vi "3D Axis Rendering.vi"(11 "rotation matrix":T29=[[1.0, 0.0, 0.0, 1.0], [0.0, 1.0, 0.0, 0.0], [0.0, 0.0, 1.0, 0.0], [0.0, 0.0, 0.0, 1.0]]) -> (3 "SceneNode out":refnum<vi>(3d-picture))   [LabVIEW 2017]
uses:
  <vilib>/Analysis/Matrix/Datatypes/RealMatrix.ctl
  <vilib>/Math Plots/3D Math Plots/3D Plot/3D Plot/Typedef/Property Cluster.ctl
  <vilib>/Math Plots/3D Math Plots/3D Plot/3D Plot/Typedef/Graph Property.ctl
  <vilib>/Math Plots/3D Math Plots/3D Plot/3D Plot/Typedef/General Property.ctl
  <vilib>/Math Plots/3D Math Plots/3D Plot/3D Plot/Typedef/View Property.ctl
  <vilib>/Math Plots/3D Math Plots/3D Plot/3D Plot/Typedef/Grid Plane.ctl
  <vilib>/Math Plots/3D Math Plots/3D Plot/3D Plot/Typedef/Light Property.ctl
  <vilib>/Math Plots/3D Math Plots/3D Plot/3D Plot/Typedef/Light Specific.ctl
  <vilib>/Math Plots/3D Math Plots/3D Plot/3D Plot/Typedef/Axis Property.ctl
  <vilib>/Math Plots/3D Math Plots/3D Plot/3D Plot/Typedef/Caption Property.ctl
  <vilib>/Math Plots/3D Math Plots/3D Plot/3D Plot/Typedef/Label Property.ctl
  <vilib>/Math Plots/3D Math Plots/3D Plot/3D Plot/Typedef/Range Property.ctl
  <vilib>/Math Plots/3D Math Plots/3D Plot/3D Plot/Typedef/Range Clusters.ctl
  <vilib>/Math Plots/3D Math Plots/3D Plot/3D Plot/Typedef/Grid Property.ctl
  <vilib>/Math Plots/3D Math Plots/3D Plot/3D Plot/Typedef/Tick Property.ctl
  <vilib>/Math Plots/3D Math Plots/3D Plot/3D Plot/Typedef/Value Pair Property.ctl
  <vilib>/Math Plots/3D Math Plots/3D Plot/3D Plot/Typedef/Value Pair Cluster.ctl
  <vilib>/Math Plots/3D Math Plots/3D Plot/3D Plot/Typedef/Format Property.ctl
  <vilib>/Math Plots/3D Math Plots/3D Plot/3D Plot/Typedef/Cursor Property Array.ctl
  <vilib>/Math Plots/3D Math Plots/3D Plot/3D Plot/Typedef/Cursor Property.ctl
  <vilib>/Math Plots/3D Math Plots/3D Plot/3D Plot/Typedef/Cursor Position.ctl
  <vilib>/Math Plots/3D Math Plots/3D Plot/3D Plot/Typedef/Cursor Point.ctl
  <vilib>/Math Plots/3D Math Plots/3D Plot/3D Plot/Typedef/Sprite Type.ctl
  <vilib>/Math Plots/3D Math Plots/3D Plot/3D Plot/Typedef/Cursor Line.ctl
  <vilib>/Math Plots/3D Math Plots/3D Plot/3D Plot/Typedef/Line Type.ctl
  <vilib>/Math Plots/3D Math Plots/3D Plot/3D Plot/Typedef/Cursor Plane.ctl
  <vilib>/Math Plots/3D Math Plots/3D Plot/3D Plot/Typedef/Cursor Text.ctl
  <vilib>/Math Plots/3D Math Plots/3D Plot/3D Plot/Typedef/Apearance Property.ctl
  <vilib>/Math Plots/3D Math Plots/3D Plot/3D Plot/Typedef/Item Visibility.ctl
  <vilib>/Math Plots/3D Math Plots/3D Plot/3D Plot/Typedef/Actual Transform.ctl
  <vilib>/picture/3D Picture Control/Object/Add Object (reference).vi
  <vilib>/picture/3D Picture Control/Object/Add Object (no reference).vi
  <vilib>/picture/3D Picture Control/Object/Create Object (name).vi
  <vilib>/picture/3D Picture Control/NI_3D Picture Control.lvlib
  <vilib>/Math Plots/3D Math Plots/3D Plot/3D Plot/3D Plot.lvclass
  <vilib>/robotics/Kinematics/NI_Kinematics.lvlib
  <vilib>/Analysis/Matrix/NI_Matrix.lvlib
panel:
  in  "Property Cluster":T1={"Graph Property"={"General Property"={"Plot Area Color"=16448250, "Fast Draw?"=TRUE, "Clip Data?"=FALSE}, "View Property"={"Projection Mode"=enum."Orthographic", "View Direction"=enum."User Defined", "User Defined View Direction"={"View Latitude"=1.0472, "View Longitude"=0.7853981, "View Distance"=2.0}}, "Grid Plane"={"Grid Plane Visible"={"Draw Grid Plane X-Y"=TRUE, "Draw Grid Plane Y-Z"=TRUE, "Draw Grid Plane X-Z"=TRUE}, "Grid Antialiasing"=TRUE, "Grid Frame Color"=0}}, "Light Property"={"Enable Lighting?"=TRUE, "Ambient Color"=16448250, "Light Array"=[{"Enable Light?"=TRUE, "Light Color"=16448250, "Light Latitude"=0.7853981, "Light Longitude"=0.7853981, "Light Distance"=10.0, "Attenuation"=enum."None"}, {"Enable Light?"=FALSE, "Light Color"=16448250, "Light Latitude"=0.785398, "Light Longitude"=0.785398, "Light Distance"=10.0, "Attenuation"=enum."None"}, {"Enable Light?"=FALSE, "Light Color"=16448250, "Light Latitude"=0.785398, "Light Longitude"=0.785398, "Light Distance"=10.0, "Attenuation"=enum."None"}, {"Enable Light?"=FALSE, "Light Color"=16448250, "Light Latitude"=0.785398, "Light Longitude"=0.785398, "Light Distance"=10.0, "Attenuation"=enum."None"}]}, "Axis Property"={"Caption Property"={"Show Caption"={"Show Normal X Caption"=TRUE, "Show Normal Y Caption"=TRUE, "Show Normal Z Caption"=TRUE, "Show Opposite X Caption"=TRUE, "Show Opposite Y Caption"=TRUE, "Show Opposite Z Caption"=TRUE}, "Caption Color"={"Caption Color X"=0, "Caption Color Y"=0, "Caption Color Z"=0}, "Caption Size"={"Caption Size X"=12, "Caption Size Y"=12, "Caption Size Z"=12}, "Caption String"={"Caption X"="X Axis", "Caption Y"="Y Axis", "Caption Z "="Z Axis"}}, "Label Property"={"Show Label"={"Show Normal X Label"=TRUE, "Show Normal Y Label"=TRUE, "Show Normal Z Label"=TRUE, "Show Opposite X Label"=TRUE, "Show Opposite Y Label"=TRUE, "Show Opposite Z Label"=TRUE}, "Label Color"={"Label Color X"=0, "Label Color Y"=0, "Label Color Z"=0}, "Label Size"={"Label Size X"=8, "Label Size Y"=8, "Labe Size Z"=8}}, "Range Property"={"Range Cluster"={"X Range"={"Max X"=10.0, "Min X"=0.0}, "Y Range"={"Max Y"=10.0, "Min Y"=0.0}, "Z Range"={"Max Z"=10.0, "Min Z"=0.0}}, "Auto Range"={"Auto Range X"=TRUE, "Auto Range Y"=TRUE, "Auto Range Z"=TRUE}, "Inverted"={"Inverted X"=FALSE, "Inverted Y"=FALSE, "Inverted Z"=FALSE}, "Logarithm"={"Logarithm X"=FALSE, "Logarithm Y"=FALSE, "Logarithm Z"=FALSE}}, "Grid Property"={"Major Grid Visible"={"Draw Major Grid X"=TRUE, "Draw Major Grid Y"=TRUE, "Draw Major Grid Z"=TRUE}, "Major Grid Color"={"Major Grid Color X"=0, "Major Grid Color Y"=0, "Major Grid Color Z"=0}, "Minor Grid Visible"={"Draw Minor Grid X"=FALSE, "Draw Minor Grid Y"=FALSE, "Draw Minor Grid Z"=FALSE}, "Minor Grid Color"={"Minor Grid Color X"=9868950, "Minor Grid Color Y"=9868950, "Minor Grid Color Z"=9868950}}, "Ticks Property"={"Major Tick Visible"={"Draw Major Tick X"=TRUE, "Draw Major Tick Y"=TRUE, "Draw Major Tick Z"=TRUE}, "Major Tick Color"={"Major Tick Color X"=0, "Major Tick Color Y"=0, "Major Tick Color Z"=0}, "Major Count"={"Major Count X"=5, "Major Count Y"=5, "Major Count Z"=5}, "Minor Tick Visible"={"Draw Minor Tick X"=TRUE, "Draw Minor Tick Y"=TRUE, "Draw Minor Tick Z"=TRUE}, "Minor Tick Color"={"Minor Tick Color X"=0, "Minor Tick Color Y"=0, "Minor Tick Color Z"=0}, "Minor Count"={"Minor Count X"=3, "Minor Count Y"=3, "Minor Count Z"=3}}}, "Value Pair Property"=[{"Value Pair Array"=[], "Show Tick"=FALSE, "Show Grid"=FALSE, " Label Mode"=enum."Name"}, {"Value Pair Array"=[], "Show Tick"=FALSE, "Show Grid"=FALSE, " Label Mode"=enum."Name"}, {"Value Pair Array"=[], "Show Tick"=FALSE, "Show Grid"=FALSE, " Label Mode"=enum."Name"}], "Format Property"=["%#.2g", "%#.2g", "%#.2g"], "Cursor Property Array"=[], "Appearance Property"={"Visibility"={"Projection Palette"=TRUE, "Color Ramp Palette"=TRUE}, "Active Index"={"Active Plot"=0, "Active Cursor"=0, "Active Axis"=enum."X-axis", "Active Value Pair"=enum."X-axis", "Active Light"=enum."Light 0"}, "Backup Data"={"Plot Name"=[]}}}
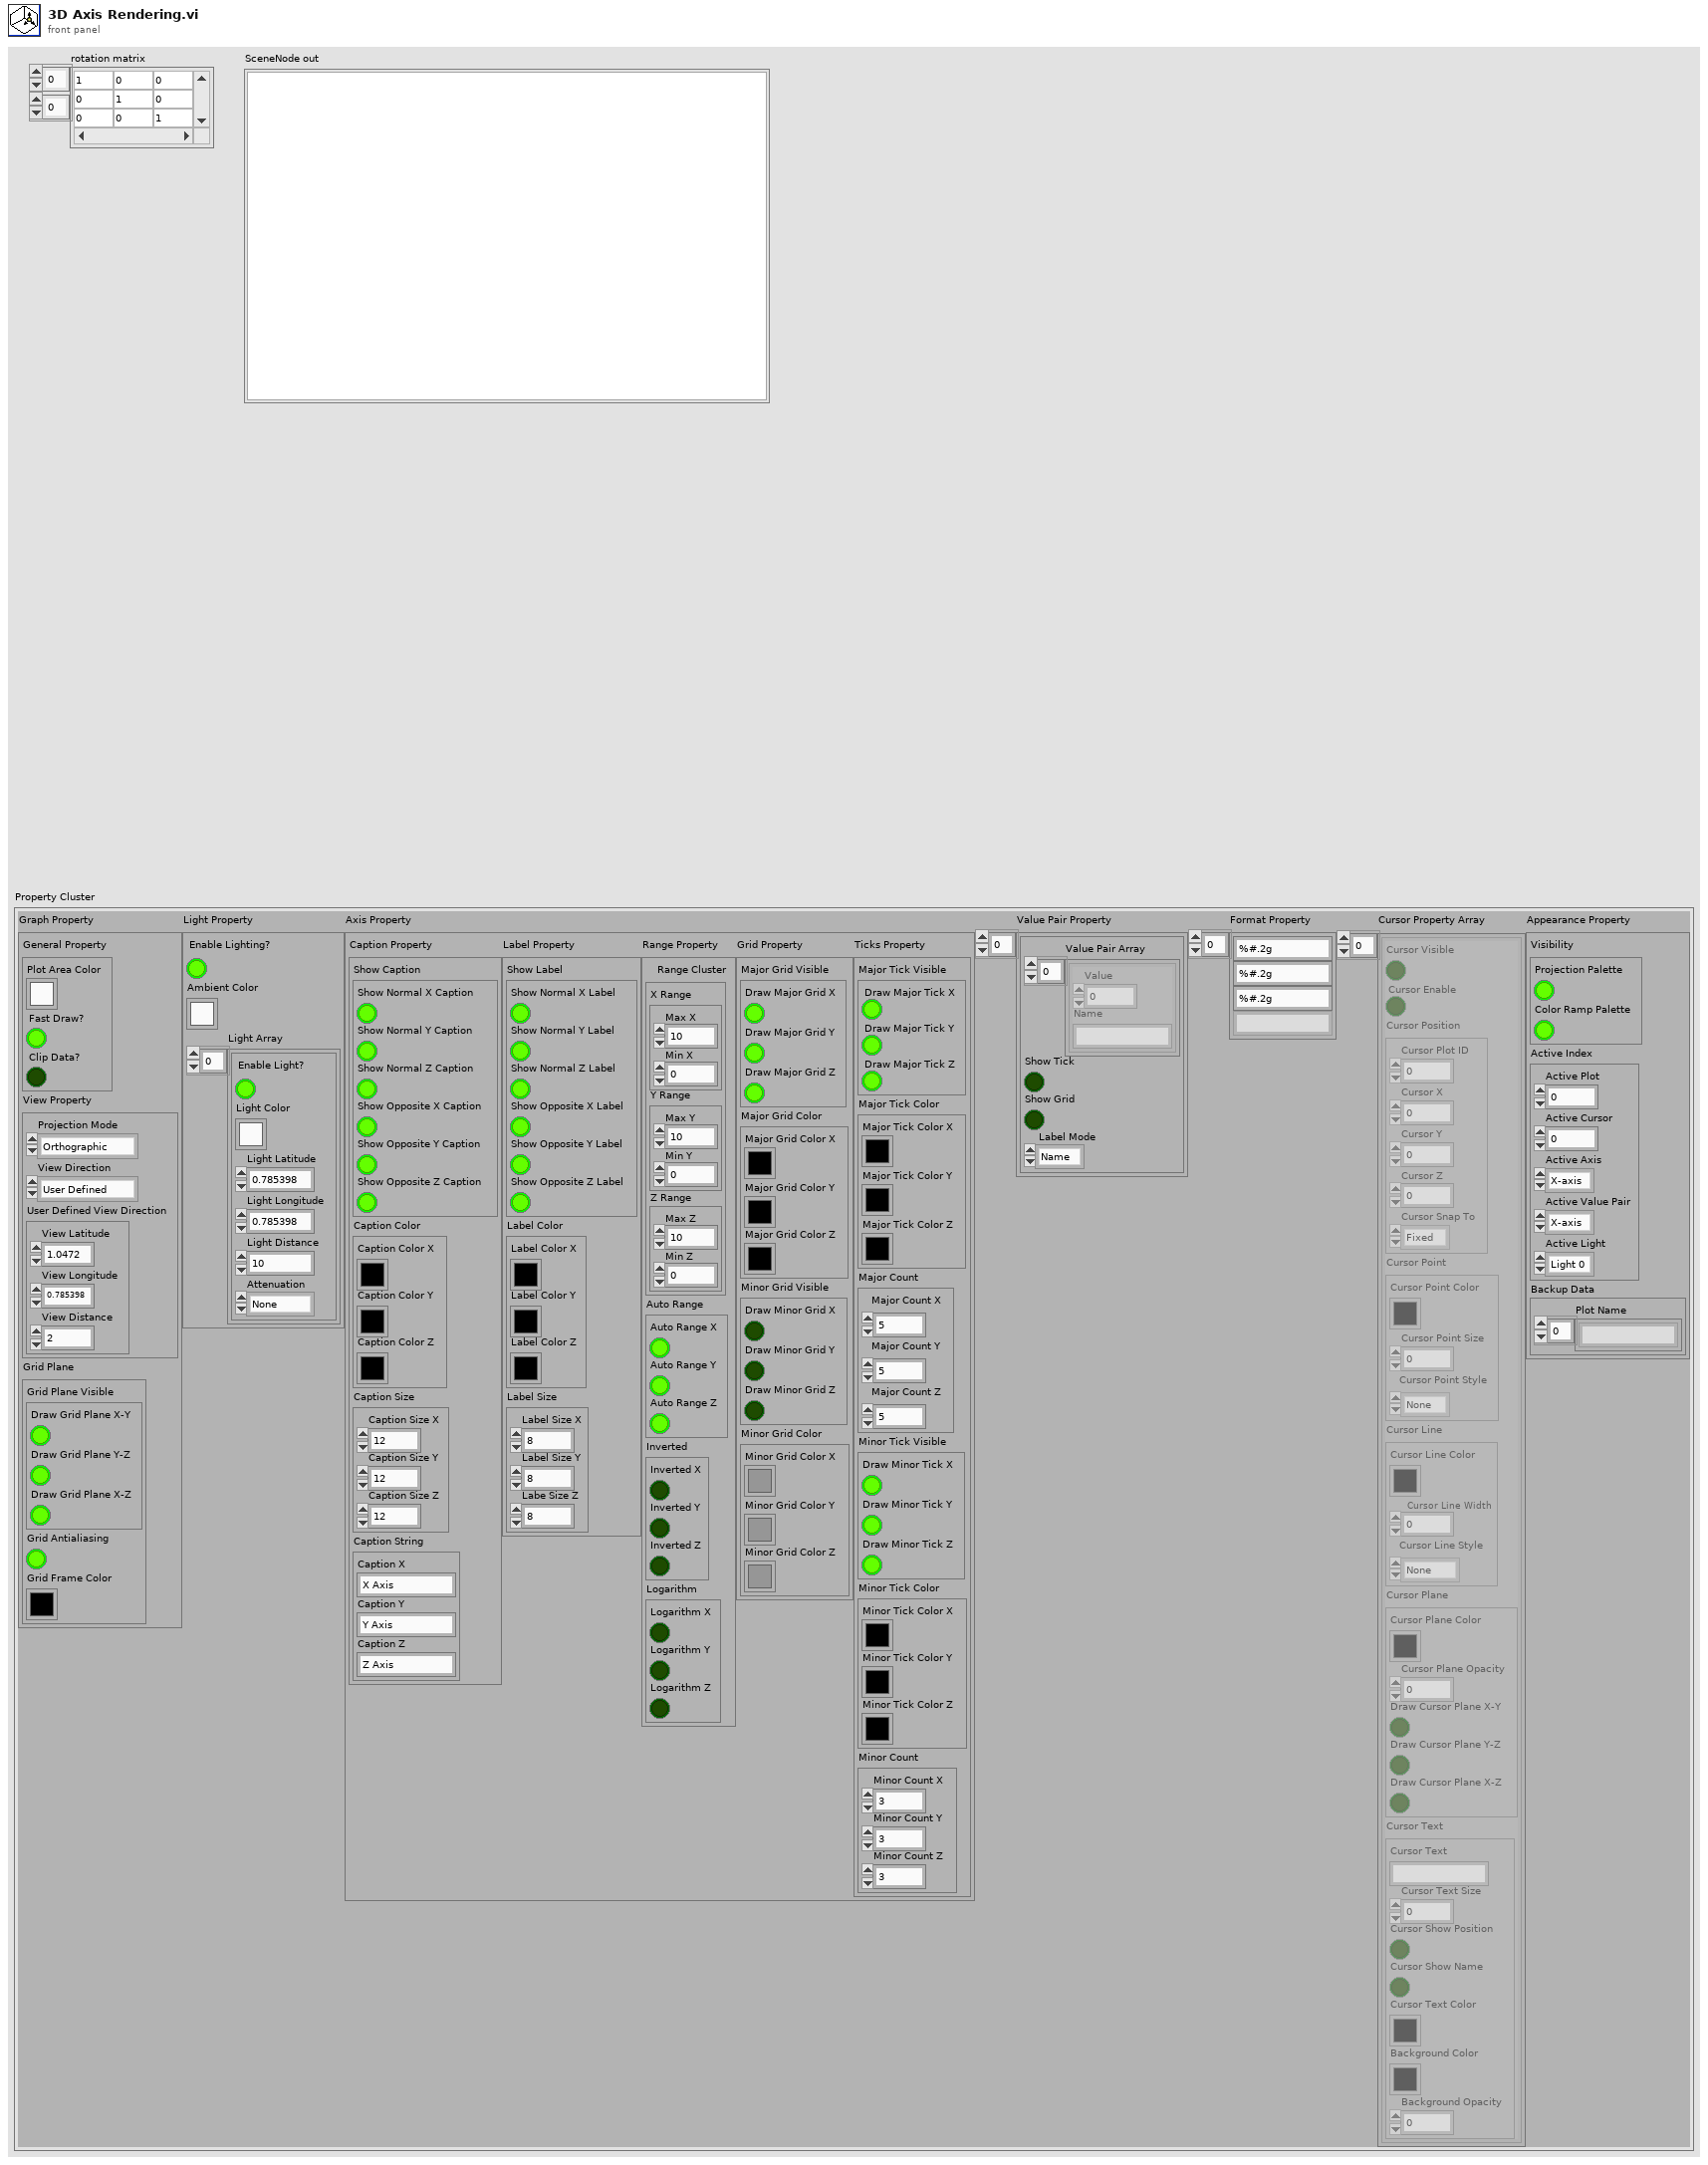
[diagram p1: front panel]
types:
  T1 = typedef "3D Plot.lvclass/Property Cluster.ctl" = cluster{"Graph Property":T2, "Light Property":T6, "Axis Property":T8, "Value Pair Property":T15, "Format Property":T17, "Cursor Property Array":T18, "Appearance Property":T27}
  T2 = typedef "3D Plot.lvclass/Graph Property.ctl" = cluster{"General Property":T3, "View Property":T4, "Grid Plane":T5}
  T3 = typedef "3D Plot.lvclass/General Property.ctl" = cluster{"Plot Area Color":u32, "Fast Draw?":bool, "Clip Data?":bool}
  T4 = typedef "3D Plot.lvclass/View Property.ctl" = cluster{"Projection Mode":enum16{"Orthographic", "Perspective"}, "View Direction":enum32{"Towards X-Y Plane", "Towards X-Z Plane", "Towards Y-Z Plane", "User Defined"}, "User Defined View Direction":cluster{"View Latitude":sgl, "View Longitude":sgl, "View Distance":sgl}}
  T5 = typedef "3D Plot.lvclass/Grid Plane.ctl" = cluster{"Grid Plane Visible":cluster{"Draw Grid Plane X-Y":bool, "Draw Grid Plane Y-Z":bool, "Draw Grid Plane X-Z":bool}, "Grid Antialiasing":bool, "Grid Frame Color":u32}
  T6 = typedef "3D Plot.lvclass/Light Property.ctl" = cluster{"Enable Lighting?":bool, "Ambient Color":u32, "Light Array":T7[]}
  T7 = typedef "3D Plot.lvclass/Light Specific.ctl" = cluster{"Enable Light?":bool, "Light Color":u32, "Light Latitude":sgl, "Light Longitude":sgl, "Light Distance":sgl, "Attenuation":enum16{"None", "Linear", "Quadratic"}}
  T8 = typedef "3D Plot.lvclass/Axis Property.ctl" = cluster{"Caption Property":T9, "Label Property":T10, "Range Property":T11, "Grid Property":T13, "Ticks Property":T14}
  T9 = typedef "3D Plot.lvclass/Caption Property.ctl" = cluster{"Show Caption":cluster{"Show Normal X Caption":bool, "Show Normal Y Caption":bool, "Show Normal Z Caption":bool, "Show Opposite X Caption":bool, "Show Opposite Y Caption":bool, "Show Opposite Z Caption":bool}, "Caption Color":cluster{"Caption Color X":u32, "Caption Color Y":u32, "Caption Color Z":u32}, "Caption Size":cluster{"Caption Size X":u16, "Caption Size Y":u16, "Caption Size Z":u16}, "Caption String":cluster{"Caption X":string, "Caption Y":string, "Caption Z ":string}}
  T10 = typedef "3D Plot.lvclass/Label Property.ctl" = cluster{"Show Label":cluster{"Show Normal X Label":bool, "Show Normal Y Label":bool, "Show Normal Z Label":bool, "Show Opposite X Label":bool, "Show Opposite Y Label":bool, "Show Opposite Z Label":bool}, "Label Color":cluster{"Label Color X":u32, "Label Color Y":u32, "Label Color Z":u32}, "Label Size":cluster{"Label Size X":u16, "Label Size Y":u16, "Labe Size Z":u16}}
  T11 = typedef "3D Plot.lvclass/Range Property.ctl" = cluster{"Range Cluster":T12, "Auto Range":cluster{"Auto Range X":bool, "Auto Range Y":bool, "Auto Range Z":bool}, "Inverted":cluster{"Inverted X":bool, "Inverted Y":bool, "Inverted Z":bool}, "Logarithm":cluster{"Logarithm X":bool, "Logarithm Y":bool, "Logarithm Z":bool}}
  T12 = typedef "3D Plot.lvclass/Range Clusters.ctl" = cluster{"X Range":cluster{"Max X":sgl, "Min X":sgl}, "Y Range":cluster{"Max Y":sgl, "Min Y":sgl}, "Z Range":cluster{"Max Z":sgl, "Min Z":sgl}}
  T13 = typedef "3D Plot.lvclass/Grid Property.ctl" = cluster{"Major Grid Visible":cluster{"Draw Major Grid X":bool, "Draw Major Grid Y":bool, "Draw Major Grid Z":bool}, "Major Grid Color":cluster{"Major Grid Color X":u32, "Major Grid Color Y":u32, "Major Grid Color Z":u32}, "Minor Grid Visible":cluster{"Draw Minor Grid X":bool, "Draw Minor Grid Y":bool, "Draw Minor Grid Z":bool}, "Minor Grid Color":cluster{"Minor Grid Color X":u32, "Minor Grid Color Y":u32, "Minor Grid Color Z":u32}}
  T14 = typedef "3D Plot.lvclass/Tick Property.ctl" = cluster{"Major Tick Visible":cluster{"Draw Major Tick X":bool, "Draw Major Tick Y":bool, "Draw Major Tick Z":bool}, "Major Tick Color":cluster{"Major Tick Color X":u32, "Major Tick Color Y":u32, "Major Tick Color Z":u32}, "Major Count":cluster{"Major Count X":u16, "Major Count Y":u16, "Major Count Z":u16}, "Minor Tick Visible":cluster{"Draw Minor Tick X":bool, "Draw Minor Tick Y":bool, "Draw Minor Tick Z":bool}, "Minor Tick Color":cluster{"Minor Tick Color X":u32, "Minor Tick Color Y":u32, "Minor Tick Color Z":u32}, "Minor Count":cluster{"Minor Count X":u16, "Minor Count Y":u16, "Minor Count Z":u16}}
  T15 = typedef "3D Plot.lvclass/Value Pair Property.ctl" = T16[]
  T16 = typedef "3D Plot.lvclass/Value Pair Cluster.ctl" = cluster{"Value Pair Array":cluster{"Value":sgl, "Name":string}[], "Show Tick":bool, "Show Grid":bool, " Label Mode":enum16{"Name", "Value", "None"}}
  T17 = typedef "3D Plot.lvclass/Format Property.ctl" = string[]
  T18 = typedef "3D Plot.lvclass/Cursor Property Array.ctl" = T19[]
  T19 = typedef "3D Plot.lvclass/Cursor Property.ctl" = cluster{"Cursor Visible":bool, "Cursor Enable":bool, "Cursor Position":T20, "Cursor Point":T21, "Cursor Line":T23, "Cursor Plane":T25, "Cursor Text":T26}
  T20 = typedef "3D Plot.lvclass/Cursor Position.ctl" = cluster{"Cursor Plot ID":i32, "Cursor X":sgl, "Cursor Y":sgl, "Cursor Z":sgl, "Cursor Snap To":enum16{"Fixed", "Nearest Plot", "Snap to Plot"}}
  T21 = typedef "3D Plot.lvclass/Cursor Point.ctl" = cluster{"Cursor Point Color":u32, "Cursor Point Size":sgl, "Cursor Point Style":T22}
  T22 = typedef "3D Plot.lvclass/Sprite Type.ctl" = enum16{"None", "Empty Square", "Solid Square", "Empty Diamond", "Solid Diamond", "Empty Circle", "Solid Circle", "Asterisk", "Bold X", "Wireframe Sphere", "Solid Sphere", "Wireframe Cube", "Solid Cube"}
  T23 = typedef "3D Plot.lvclass/Cursor Line.ctl" = cluster{"Cursor Line Color":u32, "Cursor Line Width":sgl, "Cursor Line Style":T24}
  T24 = typedef "3D Plot.lvclass/Line Type.ctl" = enum16{"None", "Solid", "Dash", "Dot", "Dash Dot"}
  T25 = typedef "3D Plot.lvclass/Cursor Plane.ctl" = cluster{"Cursor Plane Color":u32, "Cursor Plane Opacity":sgl, "Draw Cursor Plane X-Z":bool, "Draw Cursor Plane Y-Z":bool, "Draw Cursor Plane X-Y":bool}
  T26 = typedef "3D Plot.lvclass/Cursor Text.ctl" = cluster{"Cursor Text":string, "Cursor Text Size":u16, "Cursor Show Position":bool, "Cursor Show Name":bool, "Cursor Text Color":u32, "Background Color":u32, "Background Opacity":sgl}
  T27 = typedef "3D Plot.lvclass/Apearance Property.ctl" = cluster{"Visibility":T28, "Active Index":cluster{"Active Plot":i32, "Active Cursor":i32, "Active Axis":enum16{"X-axis", "Y-axis", "Z-axis"}, "Active Value Pair":enum16{"X-axis", "Y-axis", "Z-axis"}, "Active Light":enum16{"Light 0", "Light 1", "Light 2", "Light 3"}}, "Backup Data":cluster{"Plot Name":string[]}}
  T28 = typedef "3D Plot.lvclass/Item Visibility.ctl" = cluster{"Projection Palette":bool, "Color Ramp Palette":bool}
  T29 = typedef "NI_Matrix.lvlib/RealMatrix.ctl" = dbl[][]
  T30 = typedef "3D Plot.lvclass/Actual Transform.ctl" = cluster{"Scale Cluster":cluster{"X Scale":sgl, "Y Scale":sgl, "Z Scale":sgl}, "Translate Cluster":cluster{"X Translate":sgl, "Y Translate":sgl, "Z Translate":sgl}, "Actual Range":T12}
  T31 = typedef "3D Plot.lvclass/Object Cluster.ctl" = cluster{"Root Scene Object":refnum<vi>, "Fast Root Scene Object":refnum<vi>}
  T32 = cluster{"Z Translate":sgl, "Z Translate":sgl, "Z Translate":sgl}
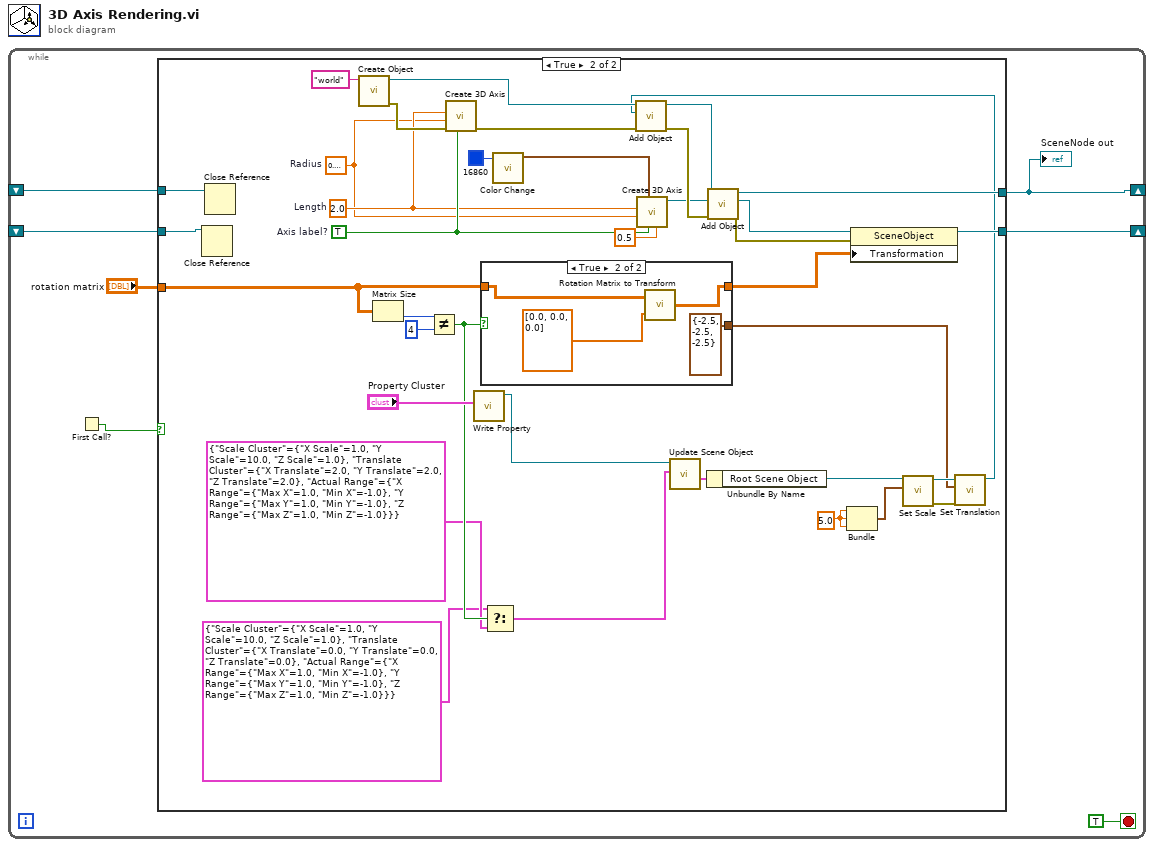
[diagram p0: block diagram]
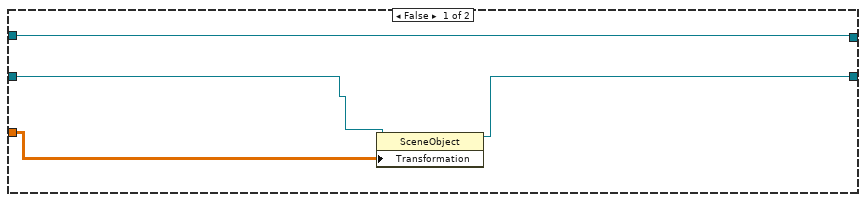
[diagram p2: hidden frame]
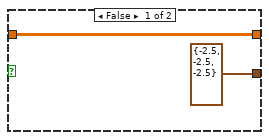
[diagram p3: hidden frame]
diagram:
  n1 = while {
    shift-right: [w5] -> _
    shift-left: _ -> [w2]
    shift-right: [w4] -> _
    shift-left: _ -> [w3]
    stop <- TRUE stop-if-true
    n2 = First Call?() -> (First Call?: T/F=w1:bool)
    n3 = case shown="True" w1 {
      tunnel: [w11 w40] -> w4
      tunnel: [w9 w27] -> w5
      tunnel: "rotation matrix" -> [w8 w23]
      tunnel: w3 -> [w11 w13]
      tunnel: w2 -> [w10 w12]
      frame False {
        n4 = property class="SceneObject"(reference=w10, "Transformation"=w8) -> (reference out=w9:refnum<vi>)  [unwired: 1 in, 1 out]
      }
      frame True {
        w33 = sgl 5.0 ("Z Translate")
        w42 = sgl 2.0  # Length
        w41 = sgl 0.1  # Radius
        w48 = TRUE  # Axis label?
        n5 = Close Reference(reference=w12) -> ()  [unwired: 1 in, 1 out]
        n6 = Close Reference(reference=w13) -> ()  [unwired: 1 in, 1 out]
        n7 = call-poly <vilib>:"Create Object.vi"("Name"="world") -> ("error out"=w44:errorcluster, "Scene:New Object"=w37:refnum<vi>)  [unwired: 9 in]
        n8 = Matrix Size(0:w23) -> (2:w25:i32)  [unwired: 1 out]
        n9 = Not Equal?(x=w25, y=4) -> (x != y?=w22:bool)
        n10 = call <vilib>:"Create 3D Axis.vi"("Axis label?"=w48, "error in (no error)"=w44, "Radius"=w41, "Length"=w42) -> ("error out"=w36:errorcluster)  [unwired: 6 in, 1 out]
        n11 = call <vilib>:"Write Property.vi"("Property Cluster"="Property Cluster") -> ("3D Plot.lvclass out"=w29:refnum<class "3D Plot.lvclass">)  [unwired: 9 in, 1 out]
        n12 = case shown="True" w22 {
          tunnel: w23 -> [w49 w54]
          tunnel: [w49 w53] -> w14
          tunnel: [cluster{"X":sgl, "Y":sgl, "Z":sgl} {"X"=-2.5, "Y"=-2.5, "Z"=-2.5} ("Translation") cluster{"X":sgl, "Y":sgl, "Z":sgl} {"X"=-2.5, "Y"=-2.5, "Z"=-2.5} ("Translation")] -> w15
          frame False {
          }
          frame True {
            n13 = call <vilib>:"Rotation Matrix to Transform.vi"("translation vector"=dbl[] [0.0, 0.0, 0.0], "rotation matrix"=w54) -> ("transform"=w53:T29)
          }
        }
        n14 = Select(t=T30 {"Scale Cluster"={"X Scale"=1.0, "Y Scale"=10.0, "Z Scale"=1.0}, "Translate Cluster"={"X Translate"=0.0, "Y Translate"=0.0, "Z Translate"=0.0}, "Actual Range"={"X Range"={"Max X"=1.0, "Min X"=-1.0}, "Y Range"={"Max Y"=1.0, "Min Y"=-1.0}, "Z Range"={"Max Z"=1.0, "Min Z"=-1.0}}} ("Actual Transform In"), s=w22, f=T30 {"Scale Cluster"={"X Scale"=1.0, "Y Scale"=10.0, "Z Scale"=1.0}, "Translate Cluster"={"X Translate"=2.0, "Y Translate"=2.0, "Z Translate"=2.0}, "Actual Range"={"X Range"={"Max X"=1.0, "Min X"=-1.0}, "Y Range"={"Max Y"=1.0, "Min Y"=-1.0}, "Z Range"={"Max Z"=1.0, "Min Z"=-1.0}}} ("Actual Transform In")) -> (s? t:f=w19:T30)
        n15 = call <vilib>:"Color Change.vi"("Color"=u32 16860) -> ("RGBA"=w46:cluster{"R":sgl, "G":sgl, "B":sgl, "A":sgl})  [unwired: 10 in]
        n16 = call <vilib>:"Create 3D Axis.vi"("Character Size"=sgl 0.5, "Axis label?"=w48, "Color"=w46, "Radius"=w41, "Length"=w42) -> ("New Object Refnum"=w31:refnum<vi>)  [unwired: 5 in, 1 out]
        n17 = call <vilib>:"Update Scene Object.vi"("Actual Transform In"=w19, "3D Plot.lvclass in"=w29) -> ("Object Cluster Out"=w35:T31)  [unwired: 5 in, 4 out]
        n18 = Unbundle By Name(w35) -> ("Root Scene Object"=w34:refnum<vi>)
        n19 = Bundle("Z Translate"=w33, "Z Translate"=w33, "Z Translate"=w33) -> (w32:T32)  [unwired: 1 in]
        n20 = call <vilib>:"Set Scale.vi"("Scale"=w32, "Scene Object"=w34) -> ("error out"=w18:errorcluster, "Scaled Object"=w17:refnum<vi>)  [unwired: 8 in]
        n21 = call <vilib>:"Set Translation.vi"("error in (no error)"=w18, "Translation"=w15, "Scene Object"=w17) -> ("Translated Object"=w16:refnum<vi>)  [unwired: 7 in, 1 out]
        n22 = call-poly <vilib>:"Add Object.vi"("error in (no error)"=w36, "New Object In"=w16, "Scene Object In"=w37) -> ("error out"=w43:errorcluster, "Scene Object Out"=w39:refnum<vi>)  [unwired: 7 in]
        n23 = call-poly <vilib>:"Add Object.vi"("error in (no error)"=w43, "New Object In"=w31, "Scene Object In"=w39) -> ("error out"=w45:errorcluster, "New Object Out"=w26:refnum<vi>, "Scene Object Out"=w40:refnum<vi>)  [unwired: 6 in]
        n24 = property class="SceneObject"(reference=w26, error in=w45, "Transformation"=w14) -> (reference out=w27:refnum<vi>)  [unwired: 1 out]
      }
    }
    "SceneNode out" <- w4
  }
